vi "Get Translation Vector.vi"(1 "transform":T1) -> (0 "translation vector":dbl[](array[numeric]))   [LabVIEW 2017, in "NI_Kinematics.lvlib"]
doc: "Returns the translation coordinates of the homogenous transform you specify.\n\n<B>.m file:</B> transl"
uses:
  <vilib>/robotics/Kinematics/NI_Kinematics.lvlib
  <vilib>/Analysis/Matrix/Datatypes/RealMatrix.ctl
  <vilib>/Analysis/Matrix/NI_Matrix.lvlib
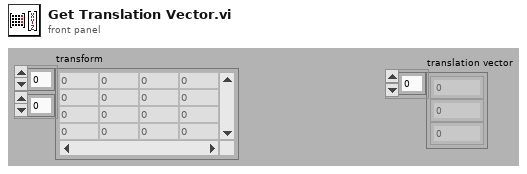
[diagram p1: front panel]
types:
  T1 = typedef "NI_Matrix.lvlib/RealMatrix.ctl" = dbl[][]
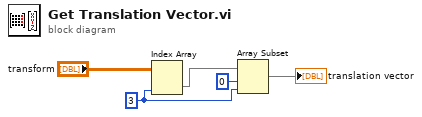
[diagram p0: block diagram]
diagram:
  w2 = 3 ("index")
  n1 = Index Array(array="transform", index (col)=w2) -> (element=w3:dbl[])  [unwired: 1 in]
  n2 = Array Subset(array=w3, index=0, length=w2) -> (→"translation vector":dbl[])
